vi "control.vi"() -> ()   [LabVIEW 2012]
uses:
  Scanning Setting.vi
panel:
  out "Scan Signal 2":cluster{"Y":dbl[], "Y":dbl[]}[](graph)
  in  "Capture":bool
  in  "DCIMG Path":path=path "H:/DATA/SET2"
  out "Frames Recorded":i32
  in  "Frames":i32=100
  out "Camera":bool=TRUE
  in  "stop":bool
  out "Image":u16[][](graph)
  in  "Snap Shut":bool
  out "Trigger":dynamicdata(graph)=[{"t0"=timestamp(16448.7 s since 1904-01-01), "dt"=1e-05, "Y"=array[10000 elements], "attributes"=variant("NI_ChannelName"=variant(string "Triangle (Collected)"), "NI_ExpIsRelativeTime"=variant(bool TRUE), "NI_ExpStartTimeStamp"=variant(timestamp timestamp(3461934223.089551 s since 1904-01-01)), "NI_ExpTimeStamp"=variant(timestamp timestamp(3461934223.089551 s since 1904-01-01)), "NI_ExpXDimension"=variant(string "t"), "NI_OriginalChannelName"=variant(string "Triangle"))}, {"t0"=timestamp(16448.7 s since 1904-01-01), "dt"=1e-05, "Y"=array[10000 elements], "attributes"=variant("NI_ChannelName"=variant(string "Square (Collected)"), "NI_ExpIsRelativeTime"=variant(bool TRUE), "NI_ExpStartTimeStamp"=variant(timestamp timestamp(3461934223.089551 s since 1904-01-01)), "NI_ExpTimeStamp"=variant(timestamp timestamp(3461934223.089551 s since 1904-01-01)), "NI_ExpXDimension"=variant(string "t"), "NI_OriginalChannelName"=variant(string "Square"))}, {"t0"=timestamp(16448.7 s since 1904-01-01), "dt"=1e-05, "Y"=array[10000 elements], "attributes"=variant("NI_ChannelName"=variant(string "Square (Collected)"), "NI_ExpIsRelativeTime"=variant(bool TRUE), "NI_ExpStartTimeStamp"=variant(timestamp timestamp(3461934223.0885506 s since 1904-01-01)), "NI_ExpTimeStamp"=variant(timestamp timestamp(3461934223.0885506 s since 1904-01-01)), "NI_ExpXDimension"=variant(string "t"), "NI_OriginalChannelName"=variant(string "Square"))}]
  out "Scan Signal":cluster{"Y":dbl[], "Y":dbl[]}[](graph)
  out "Error Out":errorcluster={"status"=TRUE, "code"=-200561, "source"="SPIM control.vi:Instance:14:1<append>\n<B>Data: </B>-10.007205\n<B>Specified Range Minimum: </B>-10.0\n<B>Specified Range Maximum: </B> 10.0\n\n<B>Task Name: </B>_unnamedTask<30>"}
  in  "Scanner":bool
  in  "Setting":bool
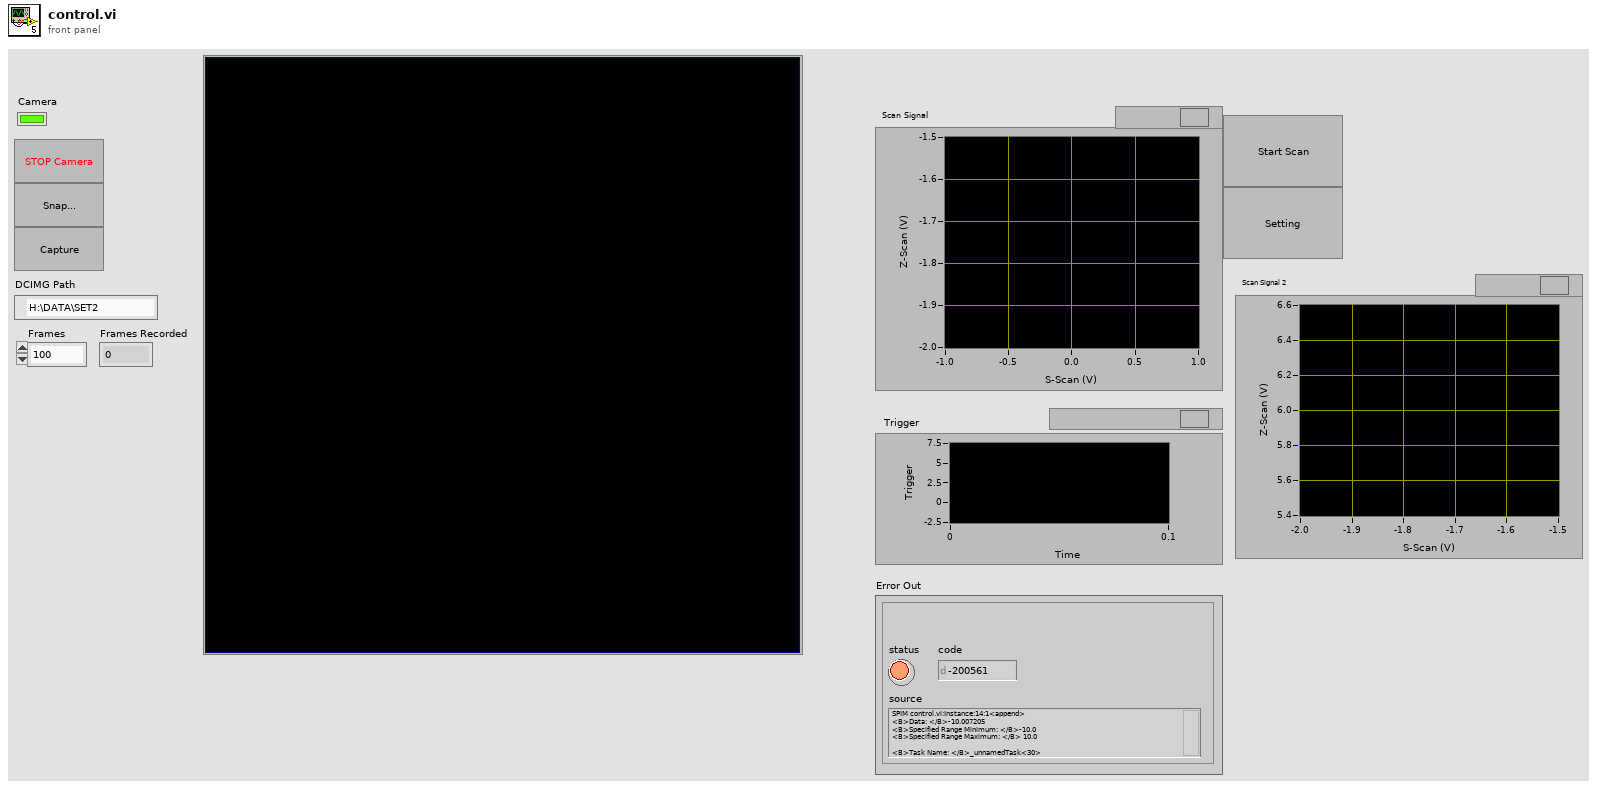
[diagram p1: front panel]
types:
  T1 = enum8{"Enabled", "Disabled", "Disabled and Grayed Out"}
  T2 = cluster{"width":u32, "height":u32, "datatype":u32}
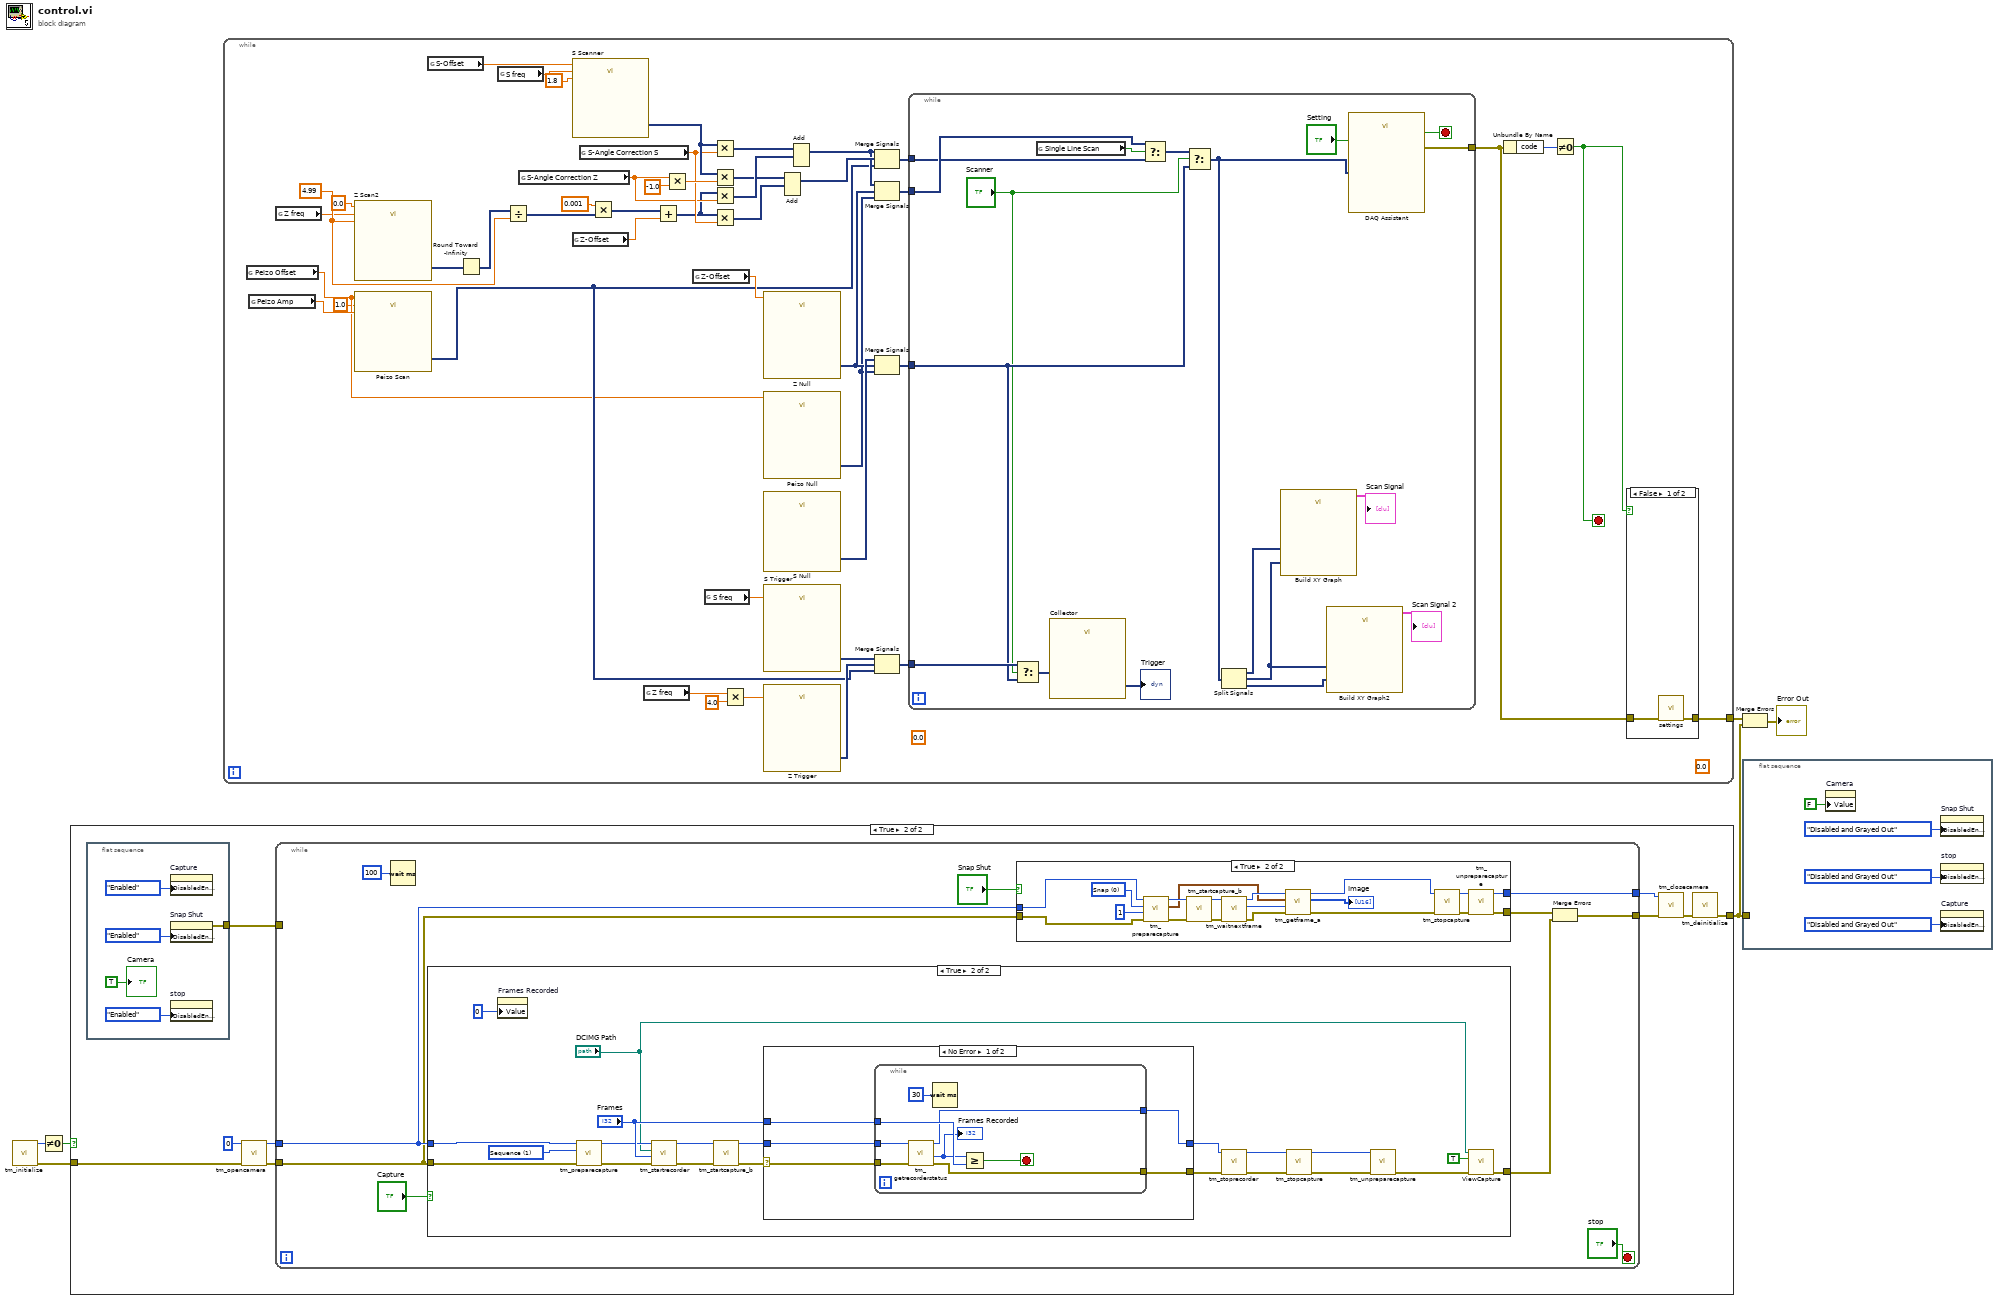
[diagram p0: block diagram]
diagram:
  n1 = call <userlib>:"tm_initialize.vi"() -> ("error out"=w3:errorcluster, "Number Of Cameras"=w4:u32)  [unwired: 10 in]
  n2 = Not Equal To 0?(x=w4) -> (x != 0?=w2:bool)
  n3 = case shown="True" w2 {
    tunnel: w3 -> [w7 w16]
    tunnel: [w7 w13] -> w1
    frame False {
    }
    frame True {
      n4 = flat-sequence {
        tunnel: [w17] -> w8
        frame #0 {
          n5 = property on="Capture" class="Bool"("DisabledEnum"=T1."Enabled" ("Disabled")) -> ()  [unwired: 2 in, 2 out]
          n6 = property on="Snap Shut" class="Bool"("DisabledEnum"=T1."Enabled" ("Disabled")) -> (error out=w17:errorcluster)  [unwired: 2 in, 1 out]
          n7 = property on="stop" class="Bool"("DisabledEnum"=T1."Enabled" ("Disabled")) -> ()  [unwired: 2 in, 2 out]
          "Camera" <- TRUE ("Camera")
        }
      }
      n8 = call <userlib>:"tm_opencamera.vi"("error in (no error)"=w16, "Camera Index"=u32 0) -> ("error out"=w9:errorcluster, "Handle out"=w10:u32)  [unwired: 8 in]
      n9 = while {
        tunnel: [w23] -> w12
        tunnel: [w31] -> w11
        tunnel: w10 -> [w27]
        tunnel: w9 -> [w26]
        tunnel: w8 -> [_]
        stop <- "stop" stop-if-true
        n10 = Wait (ms)(milliseconds to wait=u32 100) -> ()  [unwired: 1 out]
        n11 = case shown="True" "Capture" {
          tunnel: w27 -> [_ w39]
          tunnel: w26 -> [w32 w38]
          tunnel: [w32 w35] -> w25
          frame False {
          }
          frame True {
            w40 = 1 items=["Snap", "Sequence"] ("Capture mode")
            n12 = property on="Frames Recorded" class="DigNum (strict)"("Value"=0 ("Frames Recorded")) -> ()  [unwired: 2 in, 2 out]
            n13 = call <userlib>:"tm_preparecapture.vi"("error in (no error)"=w38, "Capture mode"=w40, "Handle in"=w39) -> ("error out"=w41:errorcluster, "Handle out"=w42:u32)  [unwired: 5 in, 2 out]
            n14 = call <userlib>:"tm_startrecorder.vi"("error in (no error)"=w41, "frames"="Frames", "File"="DCIMG Path", "Handle in"=w42) -> ("error out"=w43:errorcluster, "Handle out"=w44:u32)  [unwired: 6 in]
            n15 = call <userlib>:"tm_startcapture_b.vi"("error in (no error)"=w43, "Handle in"=w44) -> ("error out"=w45:errorcluster, "Handle out"=w46:u32)  [unwired: 8 in]
            n16 = case shown="No Error" w45 {
              selector: w45 -> [w58 w67]
              tunnel: w46 -> [w57 w68]
              tunnel: [w55 w68] -> w53
              tunnel: [w56 w67] -> w52
              tunnel: "Frames" -> [w54 _]
              frame No Error {
                n17 = while {
                  tunnel: w58 -> [w64]
                  tunnel: w57 -> [w63]
                  tunnel: [w62] -> w56
                  tunnel: [w65] -> w55
                  tunnel: w54 -> [w66]
                  stop <- w60 stop-if-true
                  n18 = call <userlib>:"tm_getrecorderstatus.vi"("error in (no error)"=w64, "Handle"=w63) -> ("error out"=w62:errorcluster, "Count"=w61:i32, "Handle"=w65:u32)  [unwired: 6 in, 1 out]
                  "Frames Recorded" <- w61
                  n19 = Wait (ms)(milliseconds to wait=u32 30) -> ()  [unwired: 1 out]
                  n20 = Greater Or Equal?(x=w61, y=w66) -> (x >= y?=w60:bool)
                }
              }
              frame Error {
              }
            }
            n21 = call <userlib>:"tm_stoprecorder.vi"("error in (no error)"=w52, "Handle in"=w53) -> ("error out"=w51:errorcluster, "Handle out"=w50:u32)  [unwired: 8 in]
            n22 = call <userlib>:"tm_stopcapture.vi"("error in (no error)"=w51, "Handle in"=w50) -> ("error out"=w48:errorcluster, "Handle out"=w49:u32)  [unwired: 8 in]
            n23 = call <userlib>:"tm_unpreparecapture.vi"("error in (no error)"=w48, "Handle in"=w49) -> ("error out"=w36:errorcluster)  [unwired: 8 in, 1 out]
            n24 = call "ViewCapture.vi"("error in (no error)"=w36, "Open"=TRUE, "DCIMG Path"="DCIMG Path") -> ("error out"=w35:errorcluster)  [unwired: 8 in]
          }
        }
        n25 = case shown="True" "Snap Shut" {
          tunnel: [w70 w89] -> w24
          tunnel: [w69 w88] -> w31
          tunnel: w27 -> [w69 w82]
          tunnel: w26 -> [w70 w81]
          frame False {
          }
          frame True {
            w85 = 0 items=["Snap", "Sequence"] ("Capture mode")
            n26 = call <userlib>:"tm_preparecapture.vi"("error in (no error)"=w81, "Frames"=1, "Capture mode"=w85, "Handle in"=w82) -> ("error out"=w83:errorcluster, "Buffer"=w74:T2, "Handle out"=w84:u32)  [unwired: 4 in, 1 out]
            n27 = call <userlib>:"tm_startcapture_b.vi"("error in (no error)"=w83, "Handle in"=w84) -> ("error out"=w78:errorcluster, "Handle out"=w77:u32)  [unwired: 8 in]
            n28 = call <userlib>:"tm_waitnextframe.vi"("error in (no error)"=w78, "Handle in"=w77) -> ("error out"=w76:errorcluster, "Frame Index"=w73:i32, "Handle out"=w75:u32)  [unwired: 6 in, 1 out]
            n29 = call <userlib>:"tm_getframe_a.vi"("error in (no error)"=w76, "Frame Index"=w73, "Buffer"=w74, "Handle in"=w75) -> ("error out"=w71:errorcluster, "Data 16"=→"Image":u16[][], "Handle out"=w72:u32)  [unwired: 3 in, 2 out]
            n30 = call <userlib>:"tm_stopcapture.vi"("error in (no error)"=w71, "Handle in"=w72) -> ("error out"=w86:errorcluster, "Handle out"=w87:u32)  [unwired: 8 in]
            n31 = call <userlib>:"tm_unpreparecapture.vi"("error in (no error)"=w86, "Handle in"=w87) -> ("error out"=w89:errorcluster, "Handle out"=w88:u32)  [unwired: 8 in]
          }
        }
        n32 = Merge Errors(w24, w25) -> (w23:errorcluster)
      }
      n33 = call <userlib>:"tm_closecamera.vi"("error in (no error)"=w12, "Handle in"=w11) -> ("error out"=w14:errorcluster)  [unwired: 9 in]
      n34 = call <userlib>:"tm_deinitialize.vi"("error in (no error)"=w14) -> ("error out"=w13:errorcluster)  [unwired: 10 in]
    }
  }
  n35 = while {
    tunnel: [w119] -> w6
    stop <- w104 stop-if-true
    w102 = 4.99 ("Amplitude")
    (unwired) 0.0 ("Offset")
    (unwired) 0.0 ("Offset")
    n36 = global read "Scanning Setting.vi" "Peizo Offset"() -> (w91:dbl)
    n37 = global read "Scanning Setting.vi" "Peizo Amp"() -> (w92:dbl)
    n38 = global read "Scanning Setting.vi" "Z freq"() -> (w94:dbl)
    n39 = call "Z Scan2"("Offset"=0.0, "Frequency"=w94, "Amplitude"=w102) -> ("Triangle"=w99:dynamicdata)  [unwired: 11 in, 1 out]
    n40 = call "Peizo Scan"("Offset"=w91, "Frequency"=1.0, "Amplitude"=w92) -> ("Sine"=w93:dynamicdata)  [unwired: 11 in, 1 out]
    n41 = global read "Scanning Setting.vi" "S-Offset"() -> (w122:dbl)
    n42 = Round Toward -Infinity(1:w99) -> (0:w100:dynamicdata)
    n43 = global read "Scanning Setting.vi" "S freq"() -> (w123:dbl)
    n44 = Divide(x=w100, y=w102) -> (x/y=w103:dynamicdata)
    n45 = global read "Scanning Setting.vi" "S-Angle Correction Z"() -> (w120:dbl)
    n46 = call "S Scanner"("Offset"=w122, "Frequency"=w123, "Amplitude"=1.8) -> ("Triangle"=w127:dynamicdata)  [unwired: 11 in, 1 out]
    n47 = global read "Scanning Setting.vi" "Z-Offset"() -> (w96:dbl)
    n48 = global read "Scanning Setting.vi" "S-Angle Correction S"() -> (w121:dbl)
    n49 = Multiply(x=0.001, y=w103) -> (x*y=w98:dynamicdata)
    n50 = global read "Scanning Setting.vi" "Z freq"() -> (w108:dbl)
    n51 = Add(x=w98, y=w96) -> (x+y=w97:dynamicdata)
    n52 = Multiply(x=w120, y=-1.0) -> (x*y=w126:dbl)
    n53 = global read "Scanning Setting.vi" "Z-Offset"() -> (w118:dbl)
    n54 = global read "Scanning Setting.vi" "S freq"() -> (w114:dbl)
    n55 = Multiply(x=w127, y=w121) -> (x*y=w130:dynamicdata)
    n56 = Multiply(x=w127, y=w126) -> (x*y=w128:dynamicdata)
    n57 = Multiply(x=w97, y=w120) -> (x*y=w131:dynamicdata)
    n58 = Multiply(x=w97, y=w121) -> (x*y=w129:dynamicdata)
    n59 = Multiply(x=w108, y=4.0) -> (x*y=w109:dbl)
    n60 = call "Z Null"("Offset"=w118) -> ("Square"=w117:dynamicdata)  [unwired: 13 in, 1 out]
    n61 = call "Peizo Null"("Offset"=w91) -> ("Square"=w95:dynamicdata)  [unwired: 13 in, 1 out]
    n62 = call "S Null"() -> ("Triangle"=w135:dynamicdata)  [unwired: 14 in, 1 out]
    n63 = call "S Trigger"("Frequency"=w114) -> ("Square"=w113:dynamicdata)  [unwired: 13 in, 1 out]
    n64 = call "Z Trigger"("Frequency"=w109) -> ("Square"=w112:dynamicdata)  [unwired: 13 in, 1 out]
    n65 = Add(1:w129, 2:w128) -> (0:w124:dynamicdata)  [unwired: 1 in, 1 out]
    n66 = Add(1:w131, 2:w130) -> (0:w116:dynamicdata)  [unwired: 1 in, 1 out]
    n67 = Merge Signals(w116, w124, w93) -> (w134:dynamicdata)
    n68 = Merge Signals(w116, w117, w95) -> (w115:dynamicdata)
    n69 = Merge Signals(w135, w117, w95) -> (w133:dynamicdata)
    n70 = Merge Signals(w113, w112, w93) -> (w111:dynamicdata)
    n71 = while {
      tunnel: w134 -> [w150]
      tunnel: w133 -> [w144]
      tunnel: [w154] -> w106
      tunnel: w115 -> [w152]
      tunnel: w111 -> [w146]
      stop <- w156 stop-if-true
      n72 = Select(t=w146, s="Scanner", f=w144) -> (s? t:f=w145:dynamicdata)
      n73 = global read "Scanning Setting.vi" "Single Line Scan"() -> (w151:bool)
      n74 = call "Collector"("Signals"=w145) -> ("Collected Signals"=→"Trigger":dynamicdata)  [unwired: 9 in, 1 out]
      n75 = Select(t=w152, s=w151, f=w150) -> (s? t:f=w149:dynamicdata)
      n76 = Select(t=w149, s="Scanner", f=w144) -> (s? t:f=w148:dynamicdata)
      n77 = Split Signals(w148) -> (w140:dynamicdata, w141:dynamicdata, w139:dynamicdata)  [unwired: 3 in]
      n78 = call "Build XY Graph"("Y Input"=w141, "X Input"=w140) -> ("XY Graph"=→"Scan Signal":cluster{"Y":dbl[], "Y":dbl[]}[])  [unwired: 3 in, 6 out]
      n79 = call "Build XY Graph2"("Y Input"=w139, "X Input"=w141) -> ("XY Graph"=→"Scan Signal 2":cluster{"Y":dbl[], "Y":dbl[]}[])  [unwired: 3 in, 6 out]
      n80 = call "DAQ Assistant"("data"=w148, "stop (F)"="Setting") -> ("stopped"=w156:bool, "error out"=w154:errorcluster)  [unwired: 15 in, 1 out]
    }
    n81 = Unbundle By Name(w106) -> ("code"=w105:i32)
    n82 = Not Equal To 0?(x=w105) -> (x != 0?=w104:bool)
    n83 = case shown="False" w104 {
      tunnel: [w136 w138] -> w119
      tunnel: w106 -> [w137 w138]
      frame False {
        n84 = call "settings.vi"("Error In"=w137) -> ("Error Out"=w136:errorcluster)  [unwired: 10 in]
      }
      frame True {
      }
    }
  }
  n85 = Merge Errors(w6, w1) -> (→"Error Out":errorcluster)
  n86 = flat-sequence {
    tunnel: w1 -> [_]
    frame #0 {
      n87 = property on="Camera" class="Bool (strict)"("Value"=FALSE ("Camera")) -> ()  [unwired: 2 in, 2 out]
      n88 = property on="Snap Shut" class="Bool"("DisabledEnum"=T1."Disabled and Grayed Out" ("Disabled")) -> ()  [unwired: 2 in, 2 out]
      n89 = property on="stop" class="Bool"("DisabledEnum"=T1."Disabled and Grayed Out" ("Disabled")) -> ()  [unwired: 2 in, 2 out]
      n90 = property on="Capture" class="Bool"("DisabledEnum"=T1."Disabled and Grayed Out" ("Disabled")) -> ()  [unwired: 2 in, 2 out]
    }
  }
